vi "Page URL.vi"(8 "error in (no error)":errorcluster, 11 "GodotServer in":refnum<class "GodotServer.lvclass">) -> (0 "error out":errorcluster, 2 "Page URL":string, 3 "GodotServer out":refnum<class "GodotServer.lvclass">)   [LabVIEW 2020, in "GodotLV.lvlib" / "GodotServer.lvclass"]
doc: "Generates the URL that the web app is available at. This can be passed into a WebView2 terminal or used to open a browser session.\n\nThe page will not be available until the server is activated with <b>Start Server.vi</b>"
uses:
  GodotServer.lvclass
  GodotServer.lvclass/GodotServer.ctl
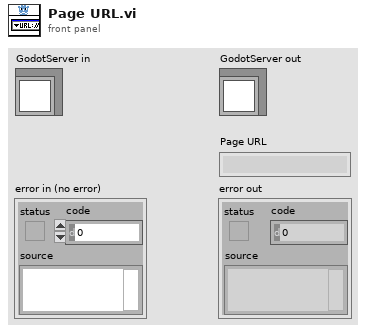
[diagram p1: front panel]
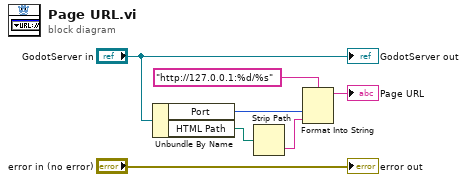
[diagram p0: block diagram]
diagram:
  n1 = Unbundle By Name("GodotServer in") -> ("Port"=w3:u16, "HTML Path"=w5:path)
  n2 = Strip Path(path=w5) -> (name=w2:string)  [unwired: 1 out]
  n3 = Format Into String(format string="http://127.0.0.1:%d/%s", w3, w2) -> (resulting string=→"Page URL":string)  [unwired: 2 in, 1 out]
  "error out" <- "error in (no error)"
  "GodotServer out" <- "GodotServer in"
